vi "Write Log Record.vi"(10 "log record":T1 {"timestamp" format="%<%x %.3X>T"}, 11 "direct handler in":refnum<class "Direct Handler.lvclass">) -> (0 "error out":errorcluster, 3 "direct handler out":refnum<class "Direct Handler.lvclass">)   [LabVIEW 2024, in "Logging.lvlib" / "Direct Handler.lvclass"]
uses:
  Direct Handler.lvclass
  Log Record.ctl
  Logger/Internal Log Levels.ctl
  Direct Handler.lvclass/Direct Handler.ctl
  Logging.lvlib
panel:
  # "Connector Pane"
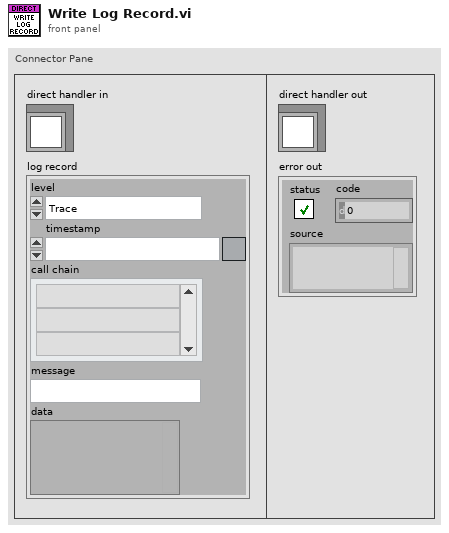
[diagram p1: front panel]
types:
  T1 = typedef "Logging.lvlib/Log Record.ctl" = cluster{"level":T2, "timestamp":timestamp, "call chain":string[], "message":string, "data":variant}
  T2 = typedef "Logging.lvlib/Internal Log Levels.ctl" = enum16{"Trace", "Debug", "Info", "Warning", "Error", "Critical", "Internal"}
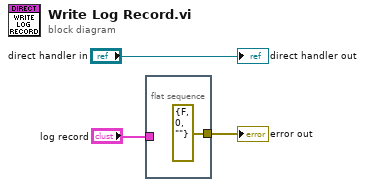
[diagram p0: block diagram]
diagram:
  n1 = flat-sequence {
    tunnel: "log record" -> [_]
    tunnel: [errorcluster {"status"=FALSE, "code"=0, "source"=""} ("error out")] -> w1
    frame #0 {
    }
  }
  "error out" <- w1
  "direct handler out" <- "direct handler in"
